vi "ubidots.vi"() -> ()   [LabVIEW 2020]
panel:
  out "error out":errorcluster
  out "concatenated string":string
  out "element 4":dbl
  out "element 3":dbl
  out "element 2":dbl
  out "element":dbl
  out "Array":dbl[](array[slide]) scale=0.0..100.0
  in  "Lim MIN T":dbl
  in  "Lim MAX T":dbl
  in  "Numeric":i32
  in  "stop":bool
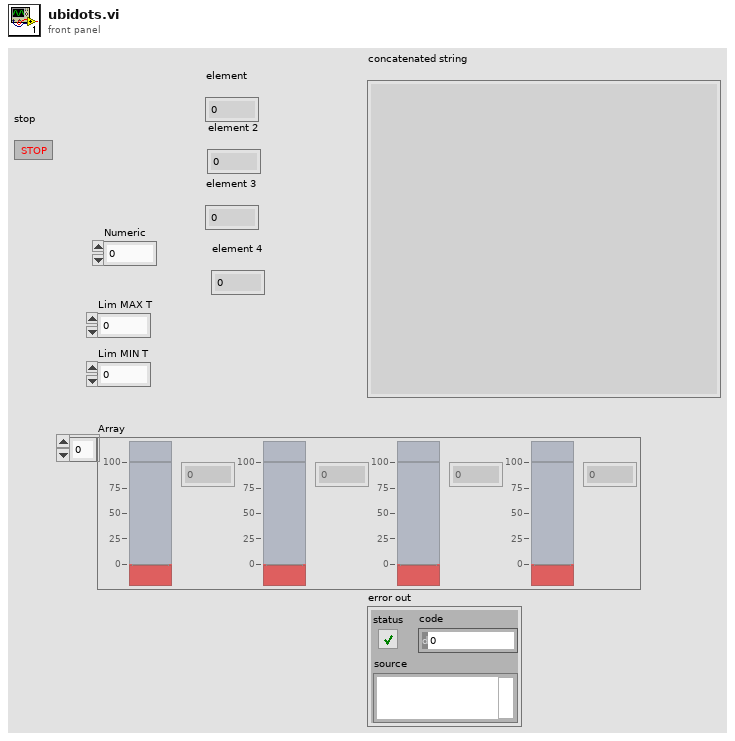
[diagram p1: front panel]
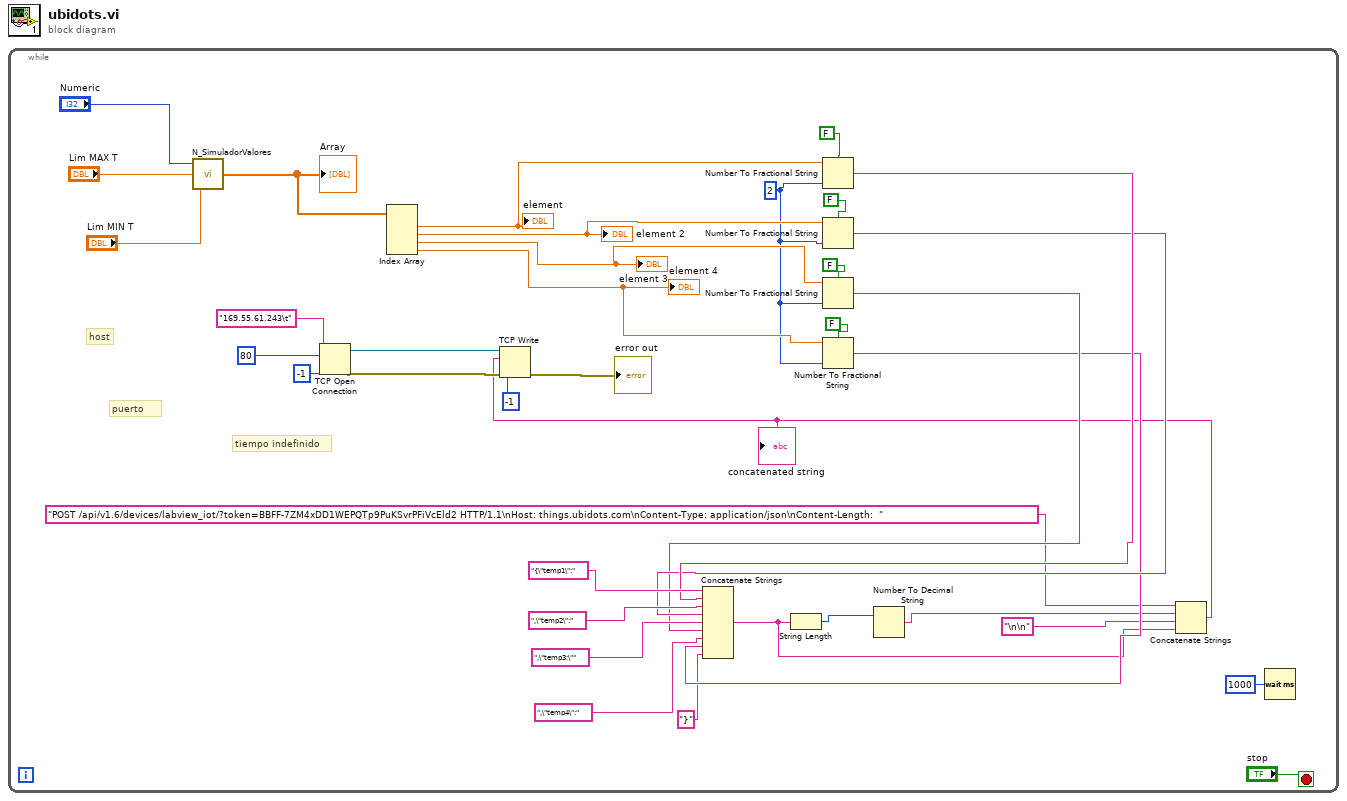
[diagram p0: block diagram]
diagram:
  n1 = while {
    stop <- "stop" stop-if-true
    w17 = 2
    # "tiempo indefinido"
    # "puerto"
    # "host"
    n2 = call "N_SimuladorValores.vi"("Lim Max T"="Lim MIN T", "Lim Min T"="Lim MAX T", "Numeric"="Numeric") -> ("Array"=w29:dbl[])
    "Array" <- w29
    n3 = TCP Open Connection(address="169.55.61.243\t", remote port or service name=u16 80, timeout ms (60000)=-1) -> (connection ID=w28:refnum<k5>, error out=w26:errorcluster)  [unwired: 2 in]
    n4 = Index Array(array=w29) -> (element #1=w21:dbl, element #2=w20:dbl, element #3=w19:dbl, element #4=w18:dbl)  [unwired: 4 in]
    "element" <- w21
    "element 2" <- w20
    "element 3" <- w19
    "element 4" <- w18
    n5 = Number To Fractional String(use system decimal point (T)=FALSE, number=w21, precision (6)=w17) -> (F-format string=w15:string)  [unwired: 1 in]
    n6 = Number To Fractional String(use system decimal point (T)=FALSE, number=w20, precision (6)=w17) -> (F-format string=w13:string)  [unwired: 1 in]
    n7 = Number To Fractional String(use system decimal point (T)=FALSE, number=w19, precision (6)=w17) -> (F-format string=w11:string)  [unwired: 1 in]
    n8 = Number To Fractional String(use system decimal point (T)=FALSE, number=w18, precision (6)=w17) -> (F-format string=w9:string)  [unwired: 1 in]
    n9 = Concatenate Strings("{\"temp1\":", w15, ",\"temp2\":", w13, ",\"temp3:\"", w11, ",\"temp4\":", w9, "}") -> (w5:string)
    n10 = String Length(string=w5) -> (length=w7:i32)
    n11 = Number To Decimal String(number=w7) -> (decimal integer string=w6:string)  [unwired: 1 in]
    n12 = Concatenate Strings("POST /api/v1.6/devices/labview_iot/?token=BBFF-7ZM4xDD1WEPQTp9PuKSvrPFiVcEld2 HTTP/1.1\nHost: things.ubidots.com\nContent-Type: application/json\nContent-Length:  " ("string"), w6, "\n\n" ("string"), w5) -> (w4:string)
    "concatenated string" <- w4
    n13 = TCP Write(connection ID=w28, data in=w4, error in (no error)=w26, 9:-1 ("timeout ms (25000)")) -> (error out=→"error out":errorcluster)  [unwired: 2 out]
    n14 = Wait (ms)(milliseconds to wait=u32 1000) -> ()  [unwired: 1 out]
  }
